vi "Set Disabled.vi"(8 "error in (no error)":errorcluster, 10 "Disabled":bool, 11 "BooleanIndicator in":refnum<class "BooleanIndicator.lvclass">) -> (0 "error out":errorcluster, 3 "BooleanIndicator out":refnum<class "BooleanIndicator.lvclass">)   [LabVIEW 2020, in "VolatusGUIElements.lvlib" / "BooleanIndicator.lvclass"]
uses:
  BooleanIndicator.lvclass
  BooleanIndicator.lvclass/BooleanIndicator.ctl
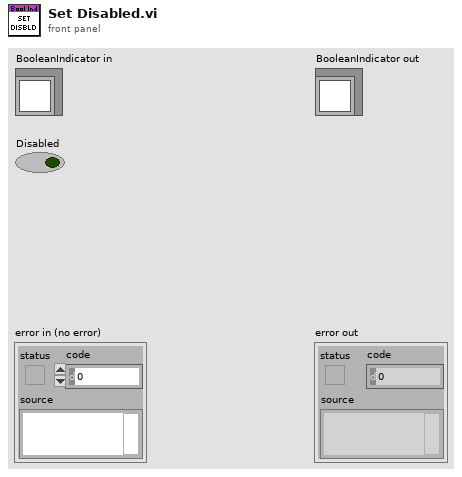
[diagram p1: front panel]
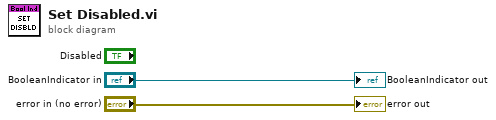
[diagram p0: block diagram]
diagram:
  "error out" <- "error in (no error)"
  "BooleanIndicator out" <- "BooleanIndicator in"
